vi "Send SMS.vi"(0 "SMTP Server":string, 1 "Carrier":enum16{"T-Mobile", "AT&T", "Verizon", "Sprint"}(ring), 3 "Phone Number":string, 5 "Email Username":string, 9 "Email Password":string, 11 "error in (no error)":errorcluster, 12 "Subject":string, 13 "Body":string, 14 "Attachments":path[](array[path])) -> (15 "error out":errorcluster)   [LabVIEW 2013]
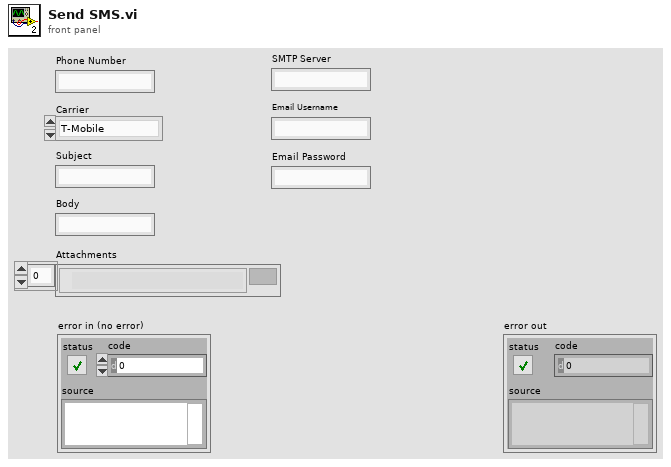
[diagram p1: front panel]
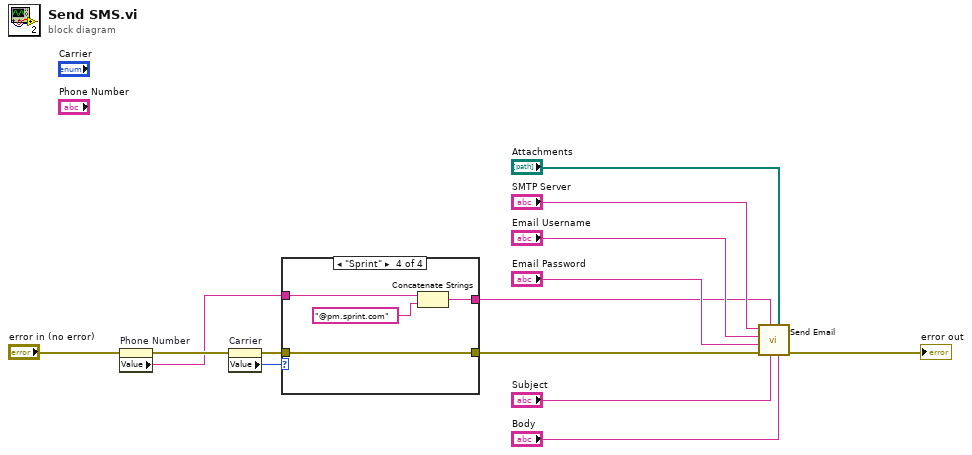
[diagram p0: block diagram]
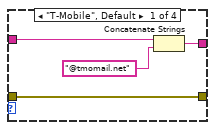
[diagram p2: hidden frame]
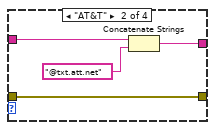
[diagram p3: hidden frame]
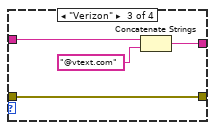
[diagram p4: hidden frame]
diagram:
  n1 = property on="Phone Number" class="Str"(error in="error in (no error)") -> (error out=w11:errorcluster, "Value"=w10:string)  [unwired: 1 in, 1 out]
  n2 = property on="Carrier" class="Enum (strict)"(error in=w11) -> (error out=w14:errorcluster, "Value"=w13:enum16{"T-Mobile", "AT&T", "Verizon", "Sprint"})  [unwired: 1 in, 1 out]
  n3 = case shown="\"Sprint\"" w13 {
    tunnel: w10 -> [w18 w21 w25 w29]
    tunnel: [w16 w22 w26 w30] -> w5
    tunnel: w14 -> [w15 w19 w23 w27]
    tunnel: [w15 w19 w23 w27] -> w9
    frame "T-Mobile", Default {
      n4 = Concatenate Strings(w18, "@tmomail.net" ("string")) -> (w16:string)
    }
    frame "AT&T" {
      n5 = Concatenate Strings(w21, "@txt.att.net" ("string")) -> (w22:string)
    }
    frame "Verizon" {
      n6 = Concatenate Strings(w25, "@vtext.com" ("string")) -> (w26:string)
    }
    frame "Sprint" {
      n7 = Concatenate Strings(w29, "@pm.sprint.com") -> (w30:string)
    }
  }
  n8 = call "Send Email.vi"("Body"="Body", "Attachments"="Attachments", "Subject"="Subject", "Email Address"=w5, "error in (no error)"=w9, "Email Password"="Email Password", "Email Username"="Email Username", "SMTP Server"="SMTP Server") -> ("error out"=→"error out":errorcluster)  [unwired: 3 in]
